vi "PI Write GPIB.vi"(0 "System no.":i32=1 min=1 max=4 step=1, 2 "String to send":string, 3 "Attach Linefeed?":bool=TRUE, 5 "error in":errorcluster) -> (19 "error out":errorcluster)   [LabVIEW 2011]
doc: "Sends command with or without trailing linefeed to selected system. \n\nValid for C-843, C-843.PM, C-844, C-848, C-865, C-880, C-880K005, E-516, E-710, E-816, F-206, M-8X0"
uses:
  E710_GCS_LabView/Low Level/Communication.llb/Global1.vi
panel:
  # "This vi sends a string w/o linefeed via the GPIB interface."
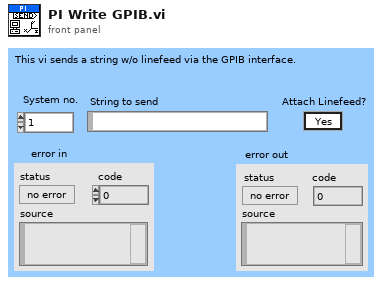
[diagram p1: front panel]
types:
  T1 = cluster{"RS232 Portnumber":u16, "Timeout":u32, "RS232 Baud rate":u32, "Interface":u16, "GPIB Bus":i32, "GPIB Address":i32, "GPIB Mode":i32}[]
  T2 = cluster{"RS232 Portnumber":u16, "Timeout":u32, "RS232 Baud rate":u32, "Interface":u16, "GPIB Bus":i32, "GPIB Address":i32, "GPIB Mode":i32}
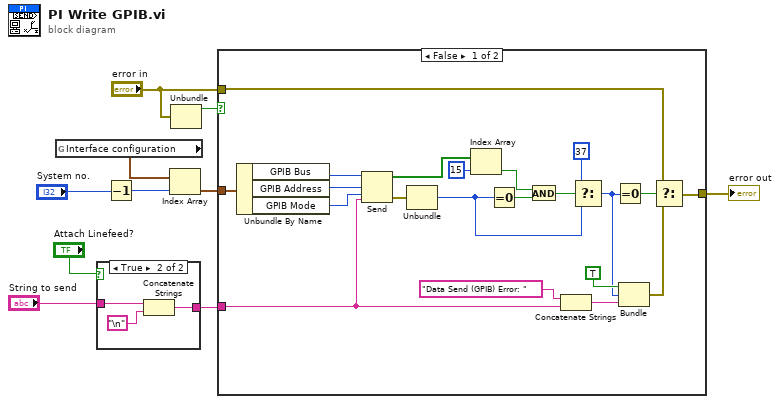
[diagram p0: block diagram]
diagram:
  n1 = global read "Global1.vi" "Interface configuration"() -> (w4:T1)
  n2 = case shown="True" "Attach Linefeed?" {
    tunnel: [w11 w14] -> w6
    tunnel: "String to send" -> [w11 w12]
    frame False {
    }
    frame True {
      n3 = Concatenate Strings(w12, "\n") -> (w14:string)
    }
  }
  n4 = Decrement(x="System no.") -> (x-1=w1:i32)
  n5 = Index Array(array=w4, index=w1) -> (element=w3:T2)
  n6 = Unbundle("error in") -> ("status"=w10:bool)  [unwired: 2 out]
  n7 = case shown="False" w10 {
    tunnel: [w18 w36] -> w8
    tunnel: "error in" -> [w20 w36]
    tunnel: w6 -> [w16 _]
    tunnel: w3 -> [w19 _]
    frame False {
      n8 = Unbundle By Name(w19) -> ("GPIB Bus"=w35:i32, "GPIB Address"=w34:i32, "GPIB Mode"=w33:i32)
      n9 = Send(0:w35, 2:w34, 3:w33, 5:w16) -> (6:w27:bool[], 8:w32:errorcluster)  [unwired: 1 in, 1 out]
      n10 = Unbundle(w32) -> ("code"=w25:i32)  [unwired: 2 out]
      n11 = Index Array(array=w27, index=15 ("Index")) -> (element=w26:bool)
      n12 = Equal To 0?(x=w25) -> (x = 0?=w28:bool)
      n13 = And(x=w26, y=w28) -> (x .and. y?=w30:bool)
      n14 = Concatenate Strings("Data Send (GPIB) Error: ", w16) -> (w15:string)
      n15 = Select(t=37, s=w30, f=w25) -> (s? t:f=w23:i32)
      n16 = Equal To 0?(x=w23) -> (x = 0?=w22:bool)
      n17 = Bundle(TRUE, "code"=w23, w15) -> (w21:cluster{bool, "code":i32, string})  [unwired: 1 in]
      n18 = Select(t=w20, s=w22, f=w21) -> (s? t:f=w18:errorcluster)
    }
    frame True {
      # "Error!"
    }
  }
  "error out" <- w8
